vi "4.4.vi"(0 "use system alert? (T)":bool=TRUE caption="使用系统警报？(T)", 1 "duration (msec)":u32 caption="持续时间（毫秒）", 2 "frequency (Hz)":u32 caption="频率(Hz)", 3 "温度":dbl) -> ()   [LabVIEW 2017]
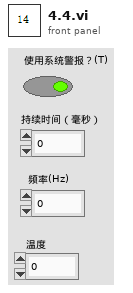
[diagram p1: front panel]
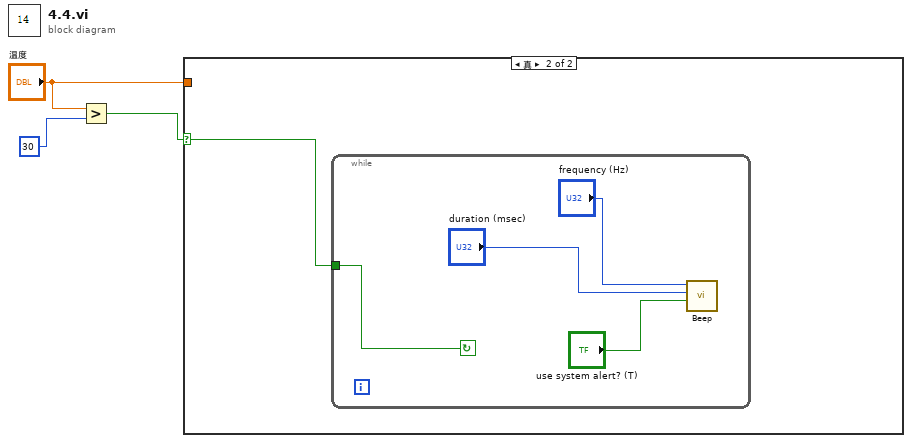
[diagram p0: block diagram]
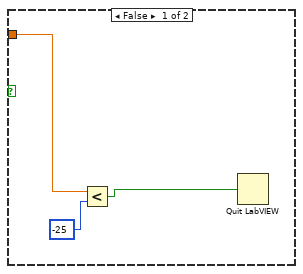
[diagram p2: hidden frame]
diagram:
  n1 = Greater?(x="温度", y=30) -> (0:w2:bool)
  n2 = case shown="真" w2 {
    selector: w2 -> [_ w7]
    tunnel: "温度" -> [w6 _]
    frame False {
      n3 = Less?(x=w6, y=-25) -> (x < y?=w4:bool)
      n4 = Quit LabVIEW(quit? (T)=w4) -> ()
    }
    frame True {
      n5 = while {
        tunnel: w7 -> [w11]
        stop <- w11 continue-if-true
        n6 = call <vilib>:"Beep.vi"("use system alert? (T)"="use system alert? (T)", "duration (msec)"="duration (msec)", "frequency (Hz)"="frequency (Hz)") -> ()  [unwired: 9 in]
      }
    }
  }
